vi "getpar1ch.vi"(4 "error in":errorcluster, 6 "value":string) -> (0 "error out":errorcluster, 2 "Cluster":T1)   [LabVIEW 2010]
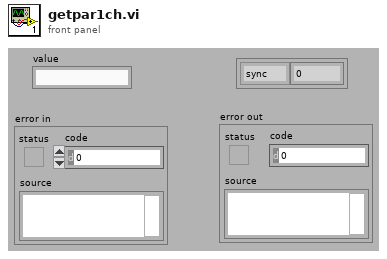
[diagram p1: front panel]
types:
  T1 = cluster{"name":enum16{"sync", "phase_a", "phase_b", "phase_c", "ground"}, "num":i32}
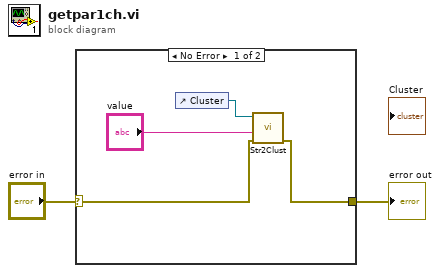
[diagram p0: block diagram]
diagram:
  n1 = case shown="No Error" "error in" {
    selector: "error in" -> [w3 w7]
    tunnel: [w6 w7] -> w2
    frame No Error {
      n2 = control-ref of="Cluster"() -> (w4:refnum<vi>)
      n3 = call "Str2Clust.vi"("error in (no error)"=w3, "String"="value", "Clust Refnum"=w4) -> ("error out"=w6:errorcluster)  [unwired: 4 in]
    }
    frame Error {
    }
  }
  "error out" <- w2
